vi "RPop.vi"(0 "reference in":refnum<class "Redis.lvclass">, 1 "Key":string, 11 "Error In":errorcluster) -> (4 "reference out":refnum<class "Redis.lvclass">, 8 "Data":T1, 15 "Error Out":errorcluster)   [LabVIEW 2020, in "Redis.lvclass"]
doc: "Removes and returns the last elements of the list stored at key."
uses:
  Redis.lvclass
  RedisDataType.ctl
  ReplyDataTypeEnum.ctl
  Redis.lvclass/Redis.ctl
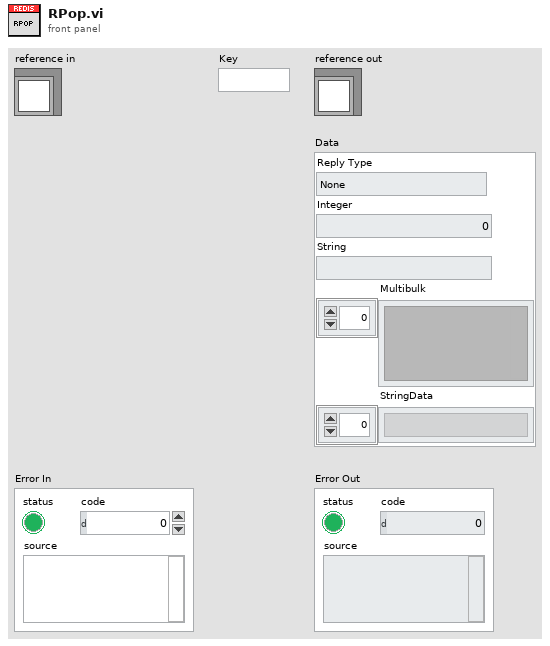
[diagram p1: front panel]
types:
  T1 = typedef "Redis.lvclass/RedisDataType.ctl" = cluster{"Reply Type":T2, "Integer":i64, "String":string, "Multibulk":variant[], "StringData":string[]}
  T2 = typedef "Redis.lvclass/ReplyDataTypeEnum.ctl" = enum16{"None", "Error", "Status", "Nil", "Integer", "String", "Multibulk"}
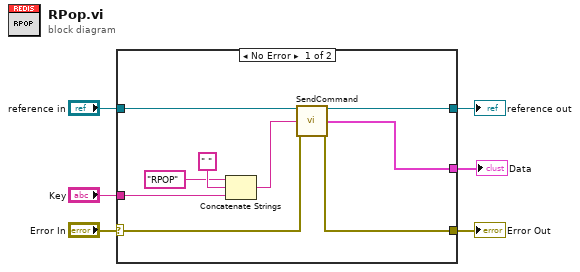
[diagram p0: block diagram]
diagram:
  n1 = case shown="No Error" "Error In" {
    selector: "Error In" -> [w13 w17]
    tunnel: [w12 w17] -> w5
    tunnel: [w15 w16] -> w3
    tunnel: "reference in" -> [w14 w16]
    tunnel: [w11 _] -> w2
    tunnel: "Key" -> [w8 _]
    frame No Error {
      n2 = Concatenate Strings("RPOP", " ", w8) -> (w7:string)
      n3 = call "SendCommand.vi"("reference in"=w14, "Command"=w7, "Error In"=w13) -> ("reference out"=w15:refnum<class "Redis.lvclass">, "Data"=w11:T1, "Error Out"=w12:errorcluster)  [unwired: 10 in]
    }
    frame Error {
    }
  }
  "Error Out" <- w5
  "reference out" <- w3
  "Data" <- w2
